vi "INIT RS232.vi"(8 "error in (no error)":errorcluster, 11 "GlobalData":T1) -> (0 "error out":errorcluster, 3 "Weight Port":refnum<visa-resource-name>)   [LabVIEW 2024]
doc: "This VI used to open RS232 Connection"
uses:
  controls/GlobalData.ctl
  <vilib>/Instr/_visa.llb/VISA Configure Serial Port (Instr).vi
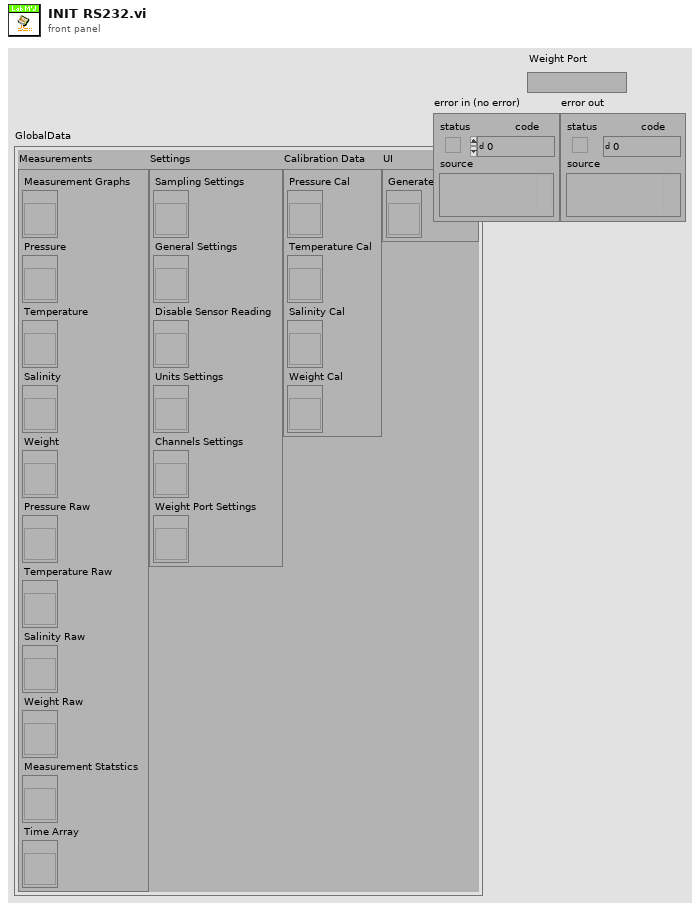
[diagram p1: front panel]
types:
  T1 = typedef "GlobalData.ctl" = cluster{"Measurements":cluster{"Measurement Graphs":refnum<vi>, "Pressure":refnum<vi>, "Temperature":refnum<vi>, "Salinity":refnum<vi>, "Weight":refnum<vi>, "Pressure Raw":refnum<vi>, "Temperature Raw":refnum<vi>, "Salinity Raw":refnum<vi>, "Weight Raw":refnum<vi>, "Measurement Statstics":refnum<vi>, "Time Array":refnum<vi>}, "Settings":cluster{"Sampling Settings":refnum<vi>, "General Settings":refnum<vi>, "Disable Sensor Reading":refnum<vi>, "Units Settings":refnum<vi>, "Channels Settings":refnum<vi>, "Weight Port Settings":refnum<vi>}, "Calibration Data":cluster{"Pressure Cal":refnum<vi>, "Temperature Cal":refnum<vi>, "Salinity Cal":refnum<vi>, "Weight Cal":refnum<vi>}, "UI":cluster{"Generate Report":refnum<vi>}}
  T2 = typedef "Serial - Settings.ctl" = cluster{"baud rate":u32, "data bits":u16, "parity":enum16{"None", "Odd", "Even", "Mark", "Space"}, "stop bits":u16, "flow control":u16}
  T3 = cluster{"Port Name":refnum<visa-resource-name>, "Port Settings":T2}
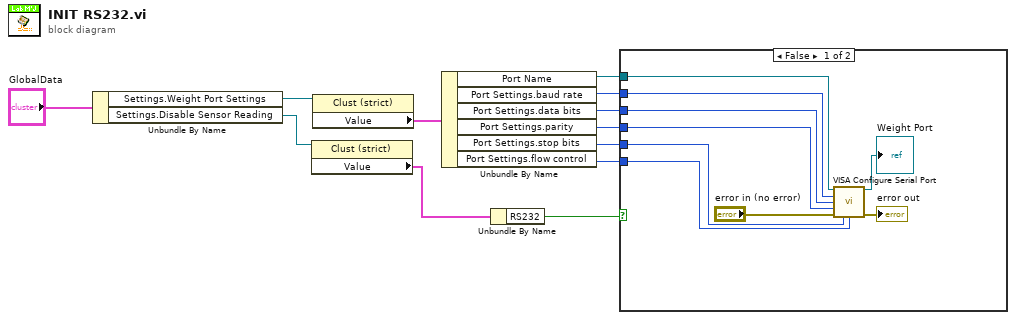
[diagram p0: block diagram]
diagram:
  n1 = Unbundle By Name("GlobalData") -> ("Settings.Weight Port Settings"=w11:refnum<vi>, "Settings.Disable Sensor Reading"=w3:refnum<vi>)
  n2 = property class="Clust (strict)"(reference=w3) -> ("Value"=w2:cluster{"Daq":bool, "RS232":bool})  [unwired: 1 in, 2 out]
  n3 = property class="Clust (strict)"(reference=w11) -> ("Value"=w10:T3)  [unwired: 1 in, 2 out]
  n4 = Unbundle By Name(w10) -> ("Port Name"=w9:refnum<visa-resource-name>, "Port Settings.baud rate"=w7:u32, "Port Settings.data bits"=w6:u16, "Port Settings.parity"=w5:enum16{"None", "Odd", "Even", "Mark", "Space"}, "Port Settings.stop bits"=w4:u16, "Port Settings.flow control"=w8:u16)
  n5 = Unbundle By Name(w2) -> ("RS232"=w1:bool)
  n6 = case shown="False" w1 {
    tunnel: w9 -> [w21 _]
    tunnel: w8 -> [w20 _]
    tunnel: w7 -> [w19 _]
    tunnel: w6 -> [w18 _]
    tunnel: w5 -> [w17 _]
    tunnel: w4 -> [w16 _]
    frame False {
      n7 = call-poly "VISA Configure Serial Port"("VISA resource name"=w21, "baud rate (9600)"=w19, "data bits (8)"=w18, "parity (0:none)"=w17, "error in (no error)"="error in (no error)", "stop bits (10: 1 bit)"=w16, "flow control (0:none)"=w20) -> ("VISA resource name out"=→"Weight Port":refnum<visa-resource-name>, "error out"=→"error out":errorcluster)  [unwired: 2 in, 5 out]
    }
    frame True {
    }
  }
